vi "Gyroscope Angle.vi"(6 "Raw Gyro Data":dbl, 8 "dt":dbl, 9 "Gyro Offset":dbl=-30.0, 10 "Previous Filtered Angle":dbl, 11 "angle HPF":dbl=0.98 format="%#_13g") -> (1 "Gyro Angle Rate":dbl, 2 "Gyro Filtered Angle":dbl, 3 "Gyro Angle":dbl(graph)=-88.01937382868523)   [LabVIEW 2014]
panel:
  in  "Gyro Divider":dbl=6545080.0 format="%#_13g"
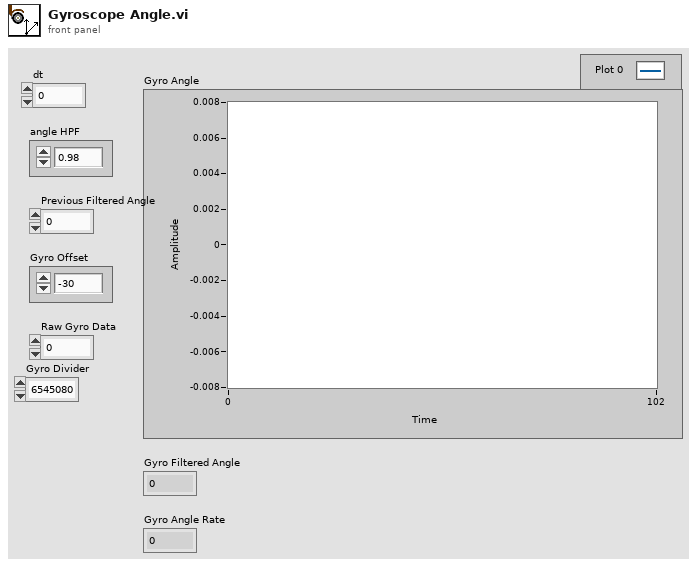
[diagram p1: front panel]
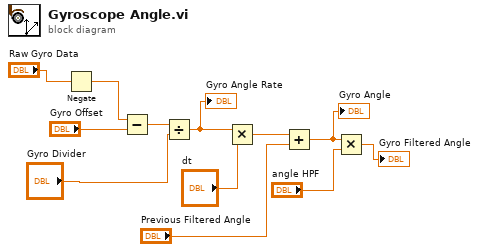
[diagram p0: block diagram]
diagram:
  n1 = Negate(x="Raw Gyro Data") -> (-x=w1:dbl)
  n2 = Subtract(x=w1, y="Gyro Offset") -> (x-y=w10:dbl)
  n3 = Divide(x=w10, y="Gyro Divider") -> (x/y=w5:dbl)
  "Gyro Angle Rate" <- w5
  n4 = Multiply(x=w5, y="dt") -> (x*y=w3:dbl)
  n5 = Add(x=w3, y="Previous Filtered Angle") -> (x+y=w12:dbl)
  "Gyro Angle" <- w12
  n6 = Multiply(x=w12, y="angle HPF") -> (x*y=→"Gyro Filtered Angle":dbl)
